vi "Show Windows System(設備運動中).vi"(8 "_error In":errorcluster, 9 "String":string, 10 "Show":bool=TRUE, 11 "vi reference in":refnum<vi>) -> (0 "_error out":errorcluster, 3 "vi reference out":refnum<vi>)   [LabVIEW 2015]
panel:
  in  "Check":bool=TRUE
  # "馬達復歸中,請稍候!"
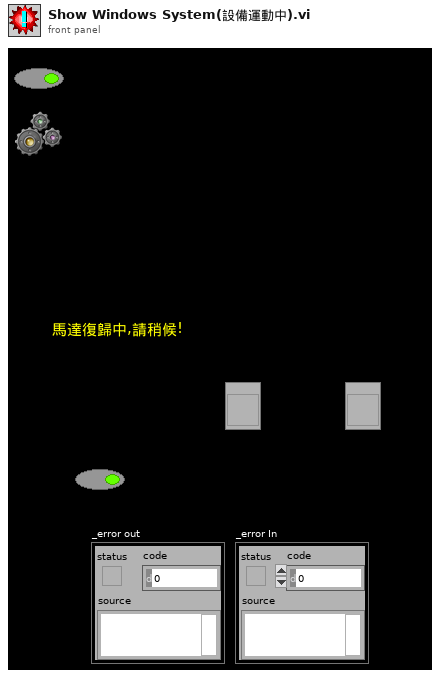
[diagram p1: front panel]
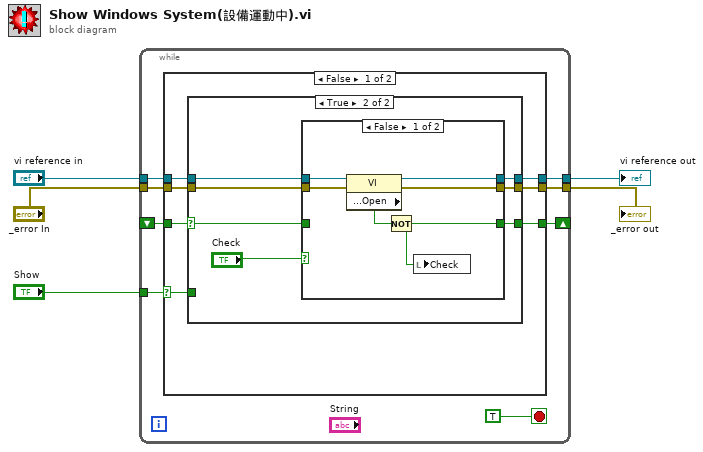
[diagram p0: block diagram]
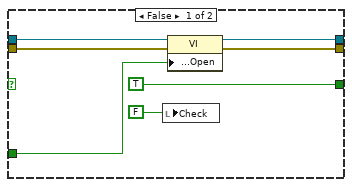
[diagram p2: hidden frame]
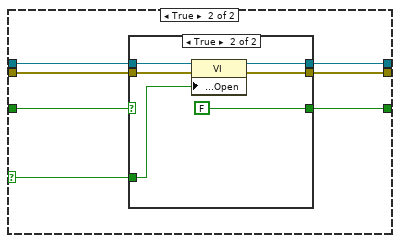
[diagram p4: hidden frame]
diagram:
  n1 = while {
    shift-right: [w9] -> _
    shift-left: _ -> [w8]
    tunnel: "Show" -> [w6]
    tunnel: "vi reference in" -> [w13]
    tunnel: "_error In" -> [w12]
    tunnel: [w11] -> w2
    tunnel: [w10] -> w1
    stop <- TRUE ("Skip Button") stop-if-true
    n2 = case shown="False" w6 {
      selector: w6 -> [w14 w44]
      tunnel: w13 -> [w20 w50]
      tunnel: w12 -> [w19 w49]
      tunnel: [w18 w48] -> w11
      tunnel: [w17 w47] -> w10
      tunnel: [w15 w46] -> w9
      tunnel: w8 -> [w16 w45]
      frame False {
        n3 = case shown="True" w16 {
          selector: w16 -> [_ w28]
          tunnel: w20 -> [w27 w34]
          tunnel: w19 -> [w26 w33]
          tunnel: [w25 w32] -> w18
          tunnel: [w24 w31] -> w17
          tunnel: [TRUE w29] -> w15
          tunnel: w14 -> [w22 _]
          frame False {
            n4 = local write "Check"(FALSE ("Check")) -> ()
            n5 = property class="VI"(reference=w27, error in=w26, "Front Panel.Open"=w22) -> (reference out=w25:refnum<vi>, error out=w24:errorcluster)
          }
          frame True {
            n6 = case shown="False" "Check" {
              tunnel: w34 -> [w40 w42]
              tunnel: w33 -> [w39 w41]
              tunnel: [w38 w42] -> w32
              tunnel: [w37 w41] -> w31
              tunnel: [w35 w43] -> w29
              tunnel: w28 -> [_ w43]
              frame False {
                n7 = property class="VI"(reference=w40, error in=w39) -> (reference out=w38:refnum<vi>, error out=w37:errorcluster, "Front Panel.Open"=w36:bool)
                n8 = Not(x=w36) -> (.not. x?=w35:bool)
                n9 = local write "Check"(w35) -> ()
              }
              frame True {
              }
            }
          }
        }
      }
      frame True {
        n10 = case shown="True" w45 {
          selector: w45 -> [w53 _]
          tunnel: w50 -> [w52 w59]
          tunnel: w49 -> [w51 w58]
          tunnel: [w52 w57] -> w48
          tunnel: [w51 w56] -> w47
          tunnel: [w53 FALSE] -> w46
          tunnel: w44 -> [_ w54]
          frame False {
          }
          frame True {
            n11 = property class="VI"(reference=w59, error in=w58, "Front Panel.Open"=w54) -> (reference out=w57:refnum<vi>, error out=w56:errorcluster)
          }
        }
      }
    }
  }
  "_error out" <- w1
  "vi reference out" <- w2
